vi "Control Fault Buses.vi"(8 "error in (no error)":errorcluster, 10 "Values":dbl[](array[numeric]), 11 "IVI Refnum in":refnum<k15>) -> (0 "error out":errorcluster, 3 "IVI Refnum out":refnum<k15>)   [LabVIEW 2020, in "PXI-2510 Engine.lvlib"]
uses:
  PXI-2510 Engine.lvlib
  <instrlib>/niSwitch/niSwitch.llb/niSwitch Relay Action.ctl
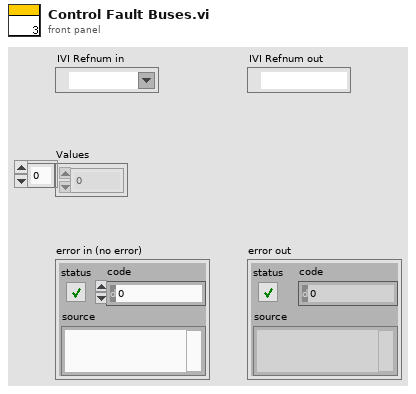
[diagram p1: front panel]
types:
  T1 = enum16{"Default", "Fault A0 to FB A", "Fault A1 to FB A", "Fault A2 to FB A", "Fault A3 to FB A", "Fault Bus A Open"}
  T2 = enum16{"Default", "Fault B0 to FB B", "Fault B1 to FB B", "Fault B2 to FB B", "Fault B3 to FB B", "Fault Bus B Open"}
  T3 = typedef "niSwitch Relay Action.ctl" = i32
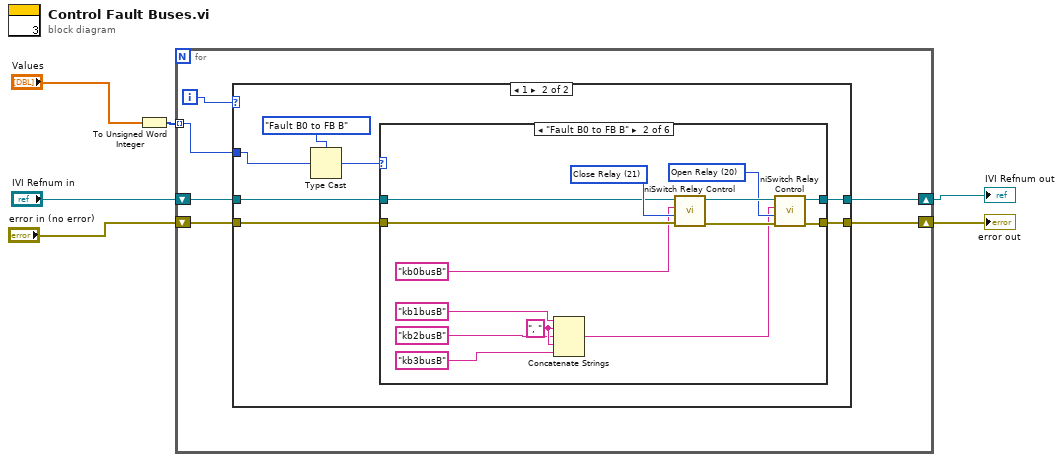
[diagram p0: block diagram]
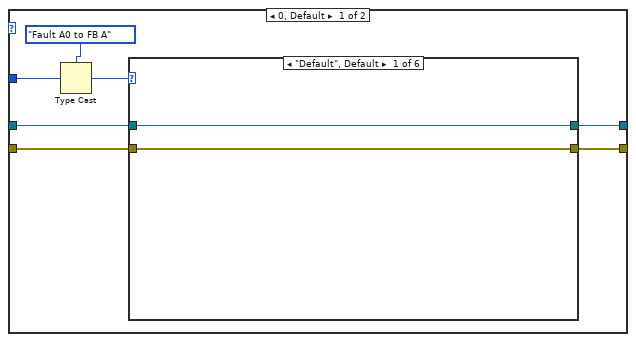
[diagram p2: hidden frame]
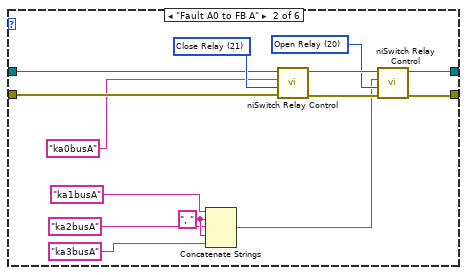
[diagram p3: hidden frame]
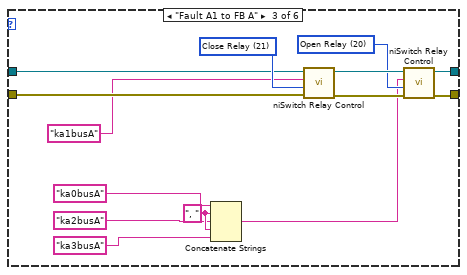
[diagram p4: hidden frame]
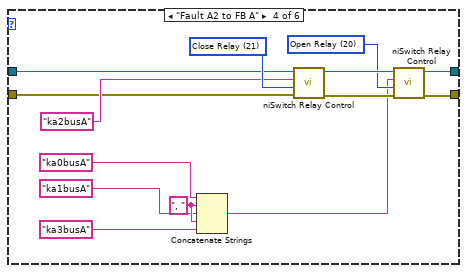
[diagram p5: hidden frame]
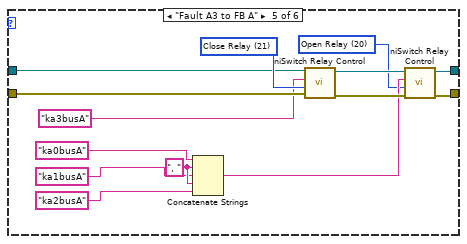
[diagram p6: hidden frame]
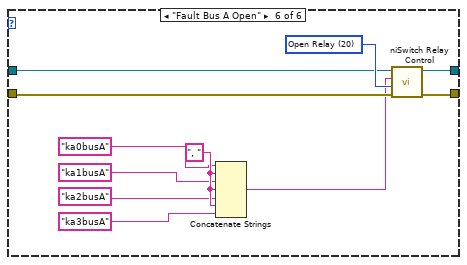
[diagram p7: hidden frame]
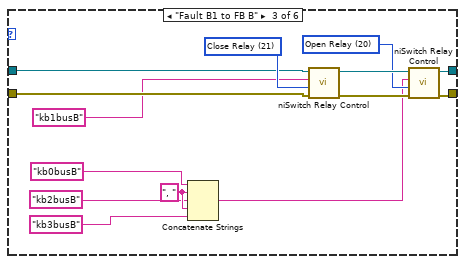
[diagram p9: hidden frame]
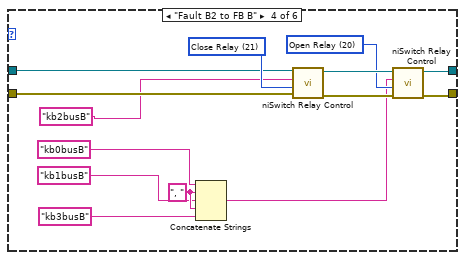
[diagram p10: hidden frame]
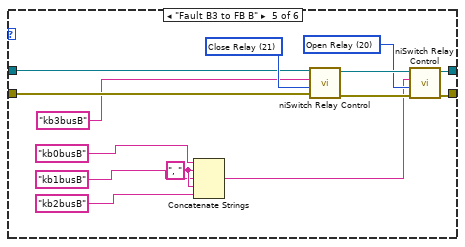
[diagram p11: hidden frame]
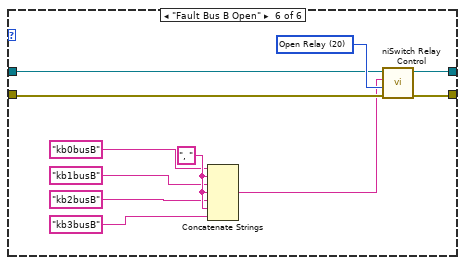
[diagram p12: hidden frame]
diagram:
  n1 = To Unsigned Word Integer(number="Values") -> (unsigned 16bit integer=w2:u16[])
  n2 = for {
    tunnel: w2 -> [w11] mode=indexing
    shift-right: [w7] -> w5
    shift-left: "IVI Refnum in" -> [w10]
    shift-right: [w8] -> w6
    shift-left: "error in (no error)" -> [w9]
    i -> [w12]
    n3 = case shown="1" w12 {
      tunnel: w11 -> [w19 w95]
      tunnel: w10 -> [w17 w92]
      tunnel: w9 -> [w16 w90]
      tunnel: [w15 w89] -> w8
      tunnel: [w14 w91] -> w7
      frame 0, Default {
        n4 = Type Cast(type=T1."Fault A0 to FB A" ("Fault Channel Operations"), x=w19) -> (*(type *) &x=w18:T1)
        n5 = case shown="\"Default\", Default" w18 {
          tunnel: w17 -> [w20 w27 w43 w53 w71 w85]
          tunnel: w16 -> [w21 w25 w42 w52 w70 w84]
          tunnel: [w21 w24 w41 w50 w69 w78] -> w15
          tunnel: [w20 w26 w40 w51 w68 w86] -> w14
          frame "Default", Default {
          }
          frame "Fault A0 to FB A" {
            w28 = T3 20 items=["Open Relay"=20, "Close Relay"=21] ("relay action (Close Relay)")
            w29 = T3 21 items=["Open Relay"=20, "Close Relay"=21] ("relay action (Close Relay)")
            w35 = ", " ("string")
            n6 = Concatenate Strings("ka1busA", w35, "ka2busA", w35, "ka3busA") -> (w23:string)
            n7 = call <instrlib>:"niSwitch Relay Control.vi"("error in (no error)"=w25, "relay action (Close Relay)"=w29, "relay names"="ka0busA", "instrument handle"=w27) -> ("error out"=w30:errorcluster, "instrument handle out"=w31:refnum<k15>)  [unwired: 6 in]
            n8 = call <instrlib>:"niSwitch Relay Control.vi"("error in (no error)"=w30, "relay action (Close Relay)"=w28, "relay names"=w23, "instrument handle"=w31) -> ("error out"=w24:errorcluster, "instrument handle out"=w26:refnum<k15>)  [unwired: 6 in]
          }
          frame "Fault A1 to FB A" {
            w45 = T3 20 items=["Open Relay"=20, "Close Relay"=21] ("relay action (Close Relay)")
            w46 = T3 21 items=["Open Relay"=20, "Close Relay"=21] ("relay action (Close Relay)")
            w49 = ", " ("string")
            n9 = Concatenate Strings("ka0busA", w49, "ka2busA", w49, "ka3busA") -> (w44:string)
            n10 = call <instrlib>:"niSwitch Relay Control.vi"("error in (no error)"=w42, "relay action (Close Relay)"=w46, "relay names"="ka1busA", "instrument handle"=w43) -> ("error out"=w47:errorcluster, "instrument handle out"=w48:refnum<k15>)  [unwired: 6 in]
            n11 = call <instrlib>:"niSwitch Relay Control.vi"("error in (no error)"=w47, "relay action (Close Relay)"=w45, "relay names"=w44, "instrument handle"=w48) -> ("error out"=w41:errorcluster, "instrument handle out"=w40:refnum<k15>)  [unwired: 6 in]
          }
          frame "Fault A2 to FB A" {
            w56 = T3 20 items=["Open Relay"=20, "Close Relay"=21] ("relay action (Close Relay)")
            w57 = T3 21 items=["Open Relay"=20, "Close Relay"=21] ("relay action (Close Relay)")
            w63 = ", " ("string")
            n12 = Concatenate Strings("ka0busA", w63, "ka1busA", w63, "ka3busA") -> (w55:string)
            n13 = call <instrlib>:"niSwitch Relay Control.vi"("error in (no error)"=w52, "relay action (Close Relay)"=w57, "relay names"="ka2busA", "instrument handle"=w53) -> ("error out"=w58:errorcluster, "instrument handle out"=w59:refnum<k15>)  [unwired: 6 in]
            n14 = call <instrlib>:"niSwitch Relay Control.vi"("error in (no error)"=w58, "relay action (Close Relay)"=w56, "relay names"=w55, "instrument handle"=w59) -> ("error out"=w50:errorcluster, "instrument handle out"=w51:refnum<k15>)  [unwired: 6 in]
          }
          frame "Fault A3 to FB A" {
            w72 = T3 20 items=["Open Relay"=20, "Close Relay"=21] ("relay action (Close Relay)")
            w74 = T3 21 items=["Open Relay"=20, "Close Relay"=21] ("relay action (Close Relay)")
            w77 = ", " ("string")
            n15 = Concatenate Strings("ka0busA", w77, "ka1busA", w77, "ka2busA") -> (w73:string)
            n16 = call <instrlib>:"niSwitch Relay Control.vi"("error in (no error)"=w70, "relay action (Close Relay)"=w74, "relay names"="ka3busA", "instrument handle"=w71) -> ("error out"=w75:errorcluster, "instrument handle out"=w76:refnum<k15>)  [unwired: 6 in]
            n17 = call <instrlib>:"niSwitch Relay Control.vi"("error in (no error)"=w75, "relay action (Close Relay)"=w72, "relay names"=w73, "instrument handle"=w76) -> ("error out"=w69:errorcluster, "instrument handle out"=w68:refnum<k15>)  [unwired: 6 in]
          }
          frame "Fault Bus A Open" {
            w87 = T3 20 items=["Open Relay"=20, "Close Relay"=21] ("relay action (Close Relay)")
            w88 = ", " ("string")
            n18 = Concatenate Strings("ka0busA", w88, "ka1busA", w88, "ka2busA", w88, "ka3busA") -> (w83:string)
            n19 = call <instrlib>:"niSwitch Relay Control.vi"("error in (no error)"=w84, "relay action (Close Relay)"=w87, "relay names"=w83, "instrument handle"=w85) -> ("error out"=w78:errorcluster, "instrument handle out"=w86:refnum<k15>)  [unwired: 6 in]
          }
        }
      }
      frame 1 {
        n20 = Type Cast(type=T2."Fault B0 to FB B" ("Fault Channel Operations"), x=w95) -> (*(type *) &x=w93:T2)
        n21 = case shown="\"Fault B0 to FB B\"" w93 {
          tunnel: w92 -> [w97 w104 w121 w133 w145 w156]
          tunnel: [w97 w106 w119 w135 w148 w158] -> w91
          tunnel: w90 -> [w96 w103 w120 w132 w144 w155]
          tunnel: [w96 w105 w118 w134 w147 w157] -> w89
          frame "Default", Default {
          }
          frame "Fault B0 to FB B" {
            w107 = T3 20 items=["Open Relay"=20, "Close Relay"=21] ("relay action (Close Relay)")
            w108 = T3 21 items=["Open Relay"=20, "Close Relay"=21] ("relay action (Close Relay)")
            w111 = ", " ("string")
            n22 = Concatenate Strings("kb1busB", w111, "kb2busB", w111, "kb3busB") -> (w102:string)
            n23 = call <instrlib>:"niSwitch Relay Control.vi"("error in (no error)"=w103, "relay action (Close Relay)"=w108, "relay names"="kb0busB", "instrument handle"=w104) -> ("error out"=w109:errorcluster, "instrument handle out"=w110:refnum<k15>)  [unwired: 6 in]
            n24 = call <instrlib>:"niSwitch Relay Control.vi"("error in (no error)"=w109, "relay action (Close Relay)"=w107, "relay names"=w102, "instrument handle"=w110) -> ("error out"=w105:errorcluster, "instrument handle out"=w106:refnum<k15>)  [unwired: 6 in]
          }
          frame "Fault B1 to FB B" {
            w117 = ", " ("string")
            w122 = T3 20 items=["Open Relay"=20, "Close Relay"=21] ("relay action (Close Relay)")
            w123 = T3 21 items=["Open Relay"=20, "Close Relay"=21] ("relay action (Close Relay)")
            n25 = Concatenate Strings("kb0busB", w117, "kb2busB", w117, "kb3busB") -> (w116:string)
            n26 = call <instrlib>:"niSwitch Relay Control.vi"("error in (no error)"=w120, "relay action (Close Relay)"=w123, "relay names"="kb1busB", "instrument handle"=w121) -> ("error out"=w124:errorcluster, "instrument handle out"=w125:refnum<k15>)  [unwired: 6 in]
            n27 = call <instrlib>:"niSwitch Relay Control.vi"("error in (no error)"=w124, "relay action (Close Relay)"=w122, "relay names"=w116, "instrument handle"=w125) -> ("error out"=w118:errorcluster, "instrument handle out"=w119:refnum<k15>)  [unwired: 6 in]
          }
          frame "Fault B2 to FB B" {
            w131 = ", " ("string")
            w136 = T3 20 items=["Open Relay"=20, "Close Relay"=21] ("relay action (Close Relay)")
            w137 = T3 21 items=["Open Relay"=20, "Close Relay"=21] ("relay action (Close Relay)")
            n28 = Concatenate Strings("kb0busB", w131, "kb1busB", w131, "kb3busB") -> (w130:string)
            n29 = call <instrlib>:"niSwitch Relay Control.vi"("error in (no error)"=w132, "relay action (Close Relay)"=w137, "relay names"="kb2busB", "instrument handle"=w133) -> ("error out"=w138:errorcluster, "instrument handle out"=w139:refnum<k15>)  [unwired: 6 in]
            n30 = call <instrlib>:"niSwitch Relay Control.vi"("error in (no error)"=w138, "relay action (Close Relay)"=w136, "relay names"=w130, "instrument handle"=w139) -> ("error out"=w134:errorcluster, "instrument handle out"=w135:refnum<k15>)  [unwired: 6 in]
          }
          frame "Fault B3 to FB B" {
            w149 = T3 20 items=["Open Relay"=20, "Close Relay"=21] ("relay action (Close Relay)")
            w150 = T3 21 items=["Open Relay"=20, "Close Relay"=21] ("relay action (Close Relay)")
            w153 = ", " ("string")
            n31 = Concatenate Strings("kb0busB", w153, "kb1busB", w153, "kb2busB") -> (w146:string)
            n32 = call <instrlib>:"niSwitch Relay Control.vi"("error in (no error)"=w144, "relay action (Close Relay)"=w150, "relay names"="kb3busB", "instrument handle"=w145) -> ("error out"=w151:errorcluster, "instrument handle out"=w152:refnum<k15>)  [unwired: 6 in]
            n33 = call <instrlib>:"niSwitch Relay Control.vi"("error in (no error)"=w151, "relay action (Close Relay)"=w149, "relay names"=w146, "instrument handle"=w152) -> ("error out"=w147:errorcluster, "instrument handle out"=w148:refnum<k15>)  [unwired: 6 in]
          }
          frame "Fault Bus B Open" {
            w159 = T3 20 items=["Open Relay"=20, "Close Relay"=21] ("relay action (Close Relay)")
            w164 = ", " ("string")
            n34 = Concatenate Strings("kb0busB", w164, "kb1busB", w164, "kb2busB", w164, "kb3busB") -> (w154:string)
            n35 = call <instrlib>:"niSwitch Relay Control.vi"("error in (no error)"=w155, "relay action (Close Relay)"=w159, "relay names"=w154, "instrument handle"=w156) -> ("error out"=w157:errorcluster, "instrument handle out"=w158:refnum<k15>)  [unwired: 6 in]
          }
        }
      }
    }
  }
  "error out" <- w6
  "IVI Refnum out" <- w5
